vi "Get VI Ref.vi"(0 "reference in":refnum<class "Generic Utilities.lvclass">, 5 "error in (no error)":errorcluster) -> (13 "VI Path":path, 14 "reference out":refnum<class "Generic Utilities.lvclass">, 17 "GUI VI Ref":refnum<vi>, 19 "error out":errorcluster)   [LabVIEW 2022 SP3, in "Generic Utilities.lvclass"]
uses:
  Generic Utilities.lvclass
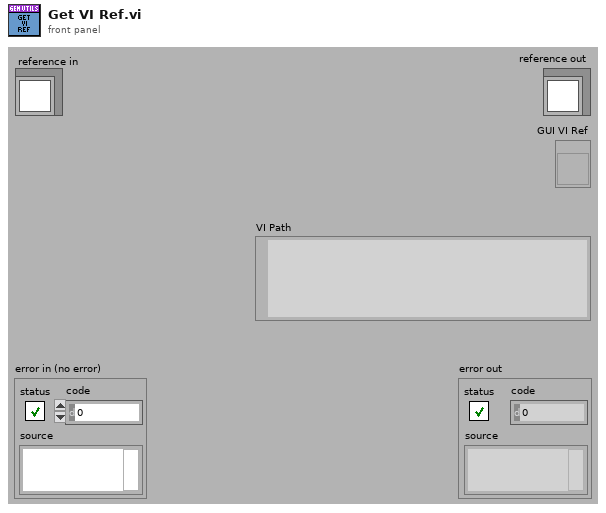
[diagram p1: front panel]
types:
  T1 = typedef "Generic Utilities.lvclass/ObjectAttributes.ctl" = cluster{"GUI Parameters":T2, "State Machine Control":cluster{"Timeout":i32, "State Queue":string[], "State History":string[], "State History Length":i32}, "Logging File Path":path, "OBJ not a refnum?":bool, "Timer Start":timestamp, "FP Refnums":T3}
  T2 = typedef "Generic Utilities.lvclass/GUI Parameters.ctl" = cluster{"Application Name":string, "GUI VI Ref":refnum<vi>, "Close Panel?":bool, "Message Window ref":refnum<vi>, "Version #":string}
  T3 = typedef "Generic Utilities.lvclass/FP Refnums.ctl" = cluster{"Panel refnum":refnum<vi>, "Control Labels":string[], "Refnums":refnum<vi>[]}
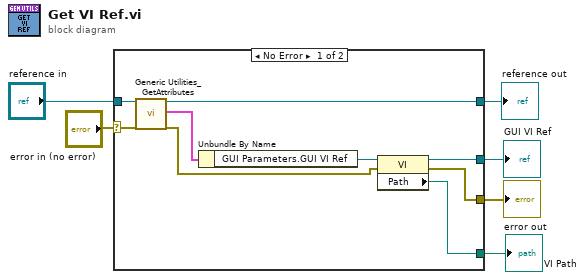
[diagram p0: block diagram]
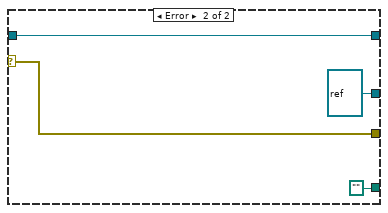
[diagram p2: hidden frame]
diagram:
  n1 = case shown="No Error" "error in (no error)" {
    selector: "error in (no error)" -> [w15 w19]
    tunnel: [w8 w19] -> w5
    tunnel: [w14 w18] -> w3
    tunnel: "reference in" -> [w12 w18]
    tunnel: [w10 refnum<vi> refnum ("GUI VI Ref")] -> w2
    tunnel: [w7 path ""] -> w1
    frame No Error {
      n2 = call "Generic Utilities_GetAttributes.vi"("reference in"=w12, "error in (no error)"=w15) -> ("reference out"=w14:refnum<class "Generic Utilities.lvclass">, "attributes"=w13:T1, "error out"=w9:errorcluster)  [unwired: 14 in, 1 out]
      n3 = Unbundle By Name(w13) -> ("GUI Parameters.GUI VI Ref"=w11:refnum<vi>)
      n4 = property class="VI"(reference=w11, error in=w9) -> (reference out=w10:refnum<vi>, error out=w8:errorcluster, "Path"=w7:path)
    }
    frame Error {
    }
  }
  "error out" <- w5
  "reference out" <- w3
  "GUI VI Ref" <- w2
  "VI Path" <- w1
